vi "Acel_calib_detector.vi"(4 "Frecuencia\nmuestreo":dbl, 5 "Pattern frequency (Hz)":dbl, 6 "Nº canales":i32, 7 "All Files in Dir":path[](array[path])) -> (0 "Continue calibrating?":bool, 1 "Reporting":string, 2 "Acceler.\ndetected":i32, 3 "Acel Cal measurements":sgl[][](array[numeric]))   [LabVIEW 2015]
uses:
  <vilib>/measure/NI_MAPro.lvlib
  <vilib>/measure/madcrms.llb/Basic Averaged DC-RMS for 1 Chan.vi
  <vilib>/Analysis/NI_AALPro.lvlib
  <vilib>/Analysis/5stat.llb/RMS (DBL).vi
panel:
  out "size(s) 3":i32
  out "size(s) 2":i32[](array[numeric])
  out "size(s)":i32[](array[numeric])
  out "element":i32
  out "max index(es)":i32
  out "max value":i32
  out "Array 3":i32[](array[numeric])
  out "sorted array":i32[](array[numeric])
  out "Array":i32[](array[numeric])
  out "OK files":bool[](array[boolean])
  out "Nº meas":i32
  out "Valid\nindex":i32[](array[numeric])
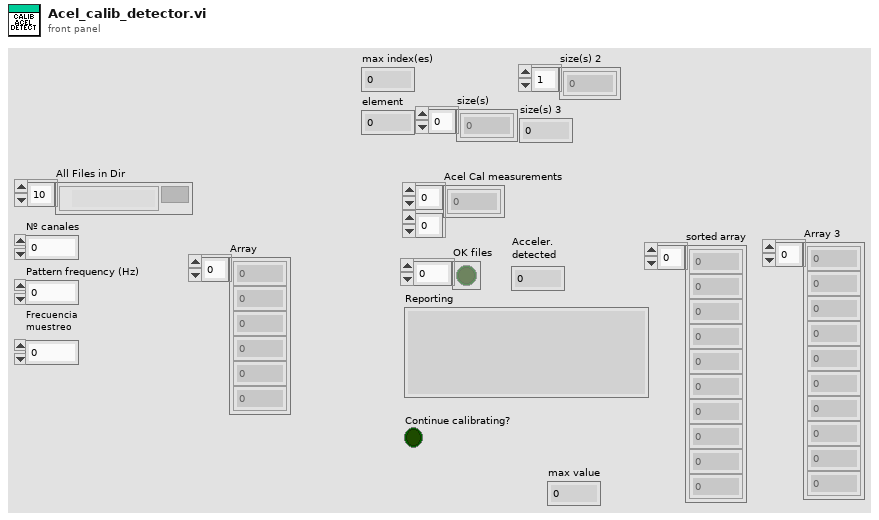
[diagram p1: front panel]
types:
  T1 = enum16{"big-endian, network order", "native, host order", "little-endian"}
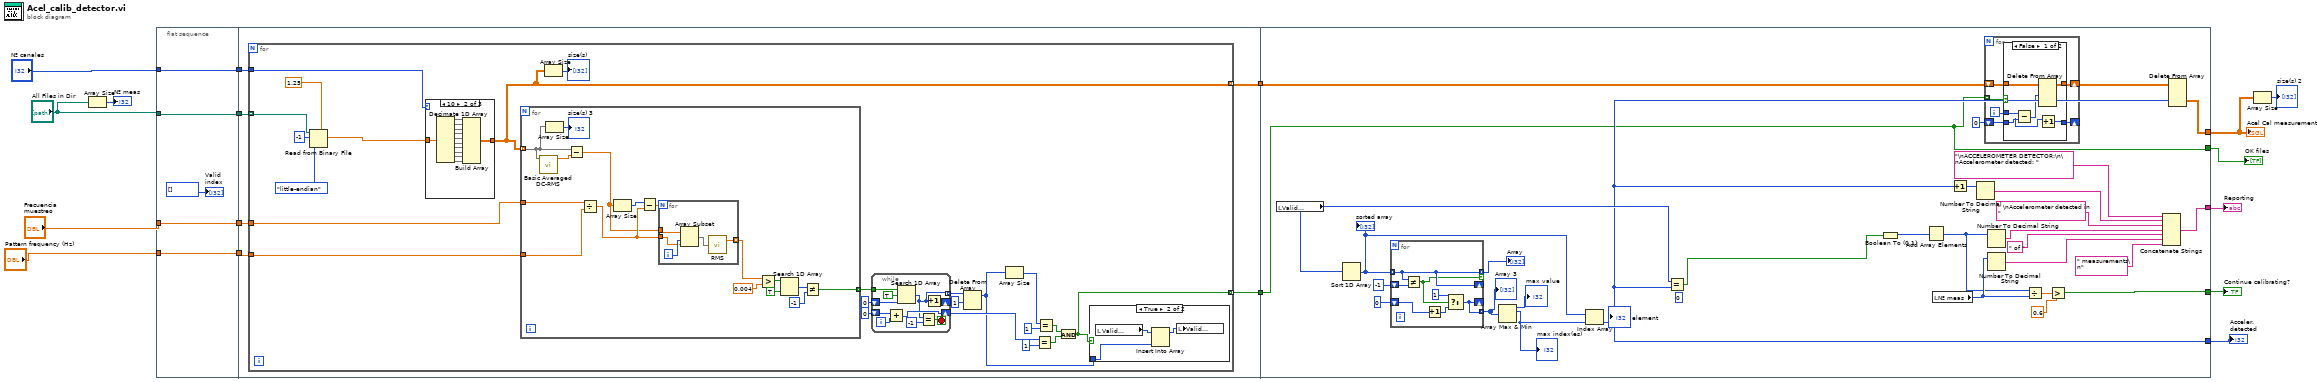
[diagram p0: block diagram]
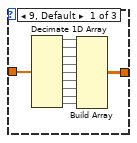
[diagram p3: hidden frame]
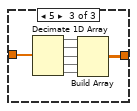
[diagram p4: hidden frame]
diagram:
  n1 = Array Size(array="All Files in Dir") -> (size(s)=→"Nº meas":i32)
  n2 = flat-sequence {
    tunnel: "All Files in Dir" -> [w21]
    tunnel: [w21] -> w17
    tunnel: [w20] -> w16
    tunnel: "Nº canales" -> [w20]
    tunnel: [w19] -> w15
    tunnel: "Frecuencia\nmuestreo" -> [w19]
    tunnel: [w18] -> w14
    tunnel: "Pattern frequency (Hz)" -> [w18]
    tunnel: [w27] -> w13
    tunnel: [w26] -> w12
    tunnel: w17 -> [w28]
    tunnel: w16 -> [w25]
    tunnel: w15 -> [w24]
    tunnel: w14 -> [w23]
    tunnel: w13 -> [w116]
    tunnel: w12 -> [w142]
    tunnel: [w141] -> w2
    tunnel: [w135] -> w4
    tunnel: [w116] -> w6
    tunnel: [w134] -> w5
    tunnel: [w121] -> w3
    frame #0 {
      "Valid\nindex" <- i32[] []
    }
    frame #1 {
      n3 = for {
        tunnel: w28 -> [w47] mode=indexing
        tunnel: [w37] -> w27 mode=indexing
        tunnel: [w30] -> w26 mode=indexing
        tunnel: w25 -> [w35]
        tunnel: w24 -> [w34]
        tunnel: w23 -> [w33]
        n4 = Read from Binary File(5:sgl 1.25, 9:T1."little-endian" ("byte order (0:big-endian, network order)"), 10:-1 ("count (1)"), 11:w47) -> (2:w48:sgl[])  [unwired: 1 in, 4 out]
        n5 = case shown="10" w35 {
          tunnel: [w65 w78 w88] -> w30
          tunnel: w48 -> [w66 w76 w89]
          frame 9, Default {
            n6 = Decimate 1D Array(w66) -> (w67:sgl[], w75:sgl[], w74:sgl[], w70:sgl[], w69:sgl[], w71:sgl[], w72:sgl[], w73:sgl[], w68:sgl[])
            n7 = Build Array(w67, w75, w74, w70, w69, w71, w72, w73, w68) -> (w65:sgl[][])
          }
          frame 10 {
            n8 = Decimate 1D Array(w76) -> (w77:sgl[], w87:sgl[], w86:sgl[], w82:sgl[], w81:sgl[], w83:sgl[], w84:sgl[], w85:sgl[], w80:sgl[], w79:sgl[])
            n9 = Build Array(w77, w87, w86, w82, w81, w83, w84, w85, w80, w79) -> (w78:sgl[][])
          }
          frame 5 {
            n10 = Decimate 1D Array(w89) -> (w90:sgl[], w94:sgl[], w93:sgl[], w92:sgl[], w91:sgl[])
            n11 = Build Array(w90, w94, w93, w92, w91) -> (w88:sgl[][])
          }
        }
        n12 = for {
          tunnel: w30 -> [w97] mode=indexing
          tunnel: [w100] -> w44 mode=indexing
          tunnel: w34 -> [w99]
          tunnel: w33 -> [w98]
          n13 = call-poly <vilib>:"Basic Averaged DC-RMS.vi"("signal in"=w97) -> ("DC value"=w110:dbl)  [unwired: 7 in, 3 out]
          n14 = Array Size(array=w97) -> (size(s)=→"size(s) 3":i32)
          n15 = Subtract(x=w97, y=w110) -> (x-y=w106:dbl[])
          n16 = Divide(x=w99, y=w98) -> (x/y=w107:dbl)
          n17 = Array Size(array=w106) -> (size(s)=w108:i32)
          n18 = Subtract(x=w108, y=w107) -> (x-y=w109:dbl)
          n19 = for {
            N: w109 -> [_]
            tunnel: w107 -> [w112]
            tunnel: [w115] -> w95 mode=indexing
            tunnel: w106 -> [w114]
            i -> [w113]
            n20 = Array Subset(array=w114, index=w113, length=w112) -> (w111:dbl[])
            n21 = call-poly <vilib>:"RMS.vi"("X"=w111) -> ("rms value"=w115:dbl)  [unwired: 1 out]
          }
          n22 = Greater?(x=w95, y=0.004 ("threshold y")) -> (0:w104:bool[])
          n23 = Search 1D Array(1D array=w104, element=TRUE) -> (index of element=w102:i32)  [unwired: 1 in]
          n24 = Not Equal?(x=w102, y=-1) -> (x != y?=w100:bool)
        }
        n25 = Array Size(array=w30) -> (size(s)=→"size(s)":i32[])
        n26 = while {
          tunnel: w44 -> [w64]
          shift-right: [w56] -> _
          shift-left: 0 ("index of element") -> [w61]
          shift-right: [w57] -> w36
          shift-left: 0 ("index of element") -> [w58]
          tunnel: [w55] -> w32 mode=indexing
          i -> [w59]
          stop <- w62 stop-if-true
          n27 = Add(x=w58, y=w59) -> (x+y=w57:i32)
          n28 = Search 1D Array(1D array=w64, element=TRUE, start index (0)=w61) -> (index of element=w55:i32)
          n29 = Equal?(x=w55, y=-1) -> (x = y?=w62:bool)
          n30 = Increment(x=w55) -> (x+1=w56:i32)
        }
        n31 = Delete From Array(array=w32, length=1) -> (array with subset deleted=w31:i32[])  [unwired: 1 in, 1 out]
        n32 = Array Size(array=w31) -> (size(s)=w40:i32)
        n33 = Equal?(x=w36, y=1) -> (x = y?=w39:bool)
        n34 = Equal?(x=w40, y=1) -> (x = y?=w38:bool)
        n35 = And(x=w38, y=w39) -> (x .and. y?=w37:bool)
        n36 = case shown="True" w37 {
          tunnel: w31 -> [_ w54]
          frame False {
          }
          frame True {
            n37 = local read "Valid\nindex"() -> (w52:i32[])
            n38 = Insert Into Array(array=w52, new element=w54) -> (w53:i32[])  [unwired: 1 in]
            n39 = local write "Valid\nindex"(w53) -> ()
          }
        }
      }
    }
    frame #2 {
      (unwired) 0 ("index of element")
      n40 = local read "Valid\nindex"() -> (w123:i32[])
      n41 = Sort 1D Array(array=w123) -> (sorted array=w117:i32[])
      "sorted array" <- w117
      n42 = for {
        tunnel: w117 -> [w151] mode=indexing
        shift-right: [w151] -> _
        shift-left: -1 ("y") -> [w152]
        tunnel: [w151] -> w128 mode=indexing if=w150
        shift-right: [w147] -> _
        shift-left: 0 ("y") -> [w148]
        tunnel: [w147] -> w126 mode=indexing
        n43 = Not Equal?(x=w151, y=w152) -> (x != y?=w150:bool)
        n44 = Increment(x=w148) -> (x+1=w149:i32)
        n45 = Select(t=1 ("y"), s=w150, f=w149) -> (s? t:f=w147:i32)
      }
      "Array" <- w128
      "Array 3" <- w126
      n46 = Array Max & Min(array=w126) -> (max value=→"max value":i32, max index (indices)=w124:i32)  [unwired: 2 out]
      "max index(es)" <- w124
      n47 = Index Array(array=w117, index=w124) -> (element=w121:i32)
      "element" <- w121
      n48 = Equal?(x=w123, y=w121) -> (x = y?=w120:bool[])
      n49 = Boolean To (0,1)(Boolean=w120) -> (0, 1=w119:i16[])
      n50 = Add Array Elements(numeric array=w119) -> (sum=w118:i16)
      n51 = local read "Nº meas"() -> (w136:i32)
      n52 = Increment(x=w121) -> (x+1=w122:i32)
      n53 = Number To Decimal String(number=w122) -> (decimal integer string=w132:string)  [unwired: 1 in]
      n54 = for {
        tunnel: w116 -> [w157] mode=indexing
        shift-right: [w156] -> w140
        shift-left: w142 -> [w158]
        shift-right: [w153] -> _
        shift-left: 0 ("index of element") -> [w154]
        i -> [w155]
        n55 = case shown="False" w157 {
          tunnel: w158 -> [w164 w166]
          tunnel: [w163 w166] -> w156
          tunnel: w155 -> [w162 _]
          tunnel: w154 -> [w159 w165]
          tunnel: [w160 w165] -> w153
          frame False {
            n56 = Subtract(x=w162, y=w159) -> (x-y=w161:i32)
            n57 = Delete From Array(array=w164, index (dim 0)=w161) -> (array with subset deleted=w163:sgl[][][])  [unwired: 3 in, 1 out]
            n58 = Increment(x=w159) -> (x+1=w160:i32)
          }
          frame True {
          }
        }
      }
      n59 = Number To Decimal String(number=w118) -> (decimal integer string=w145:string)  [unwired: 1 in]
      n60 = Number To Decimal String(number=w136) -> (decimal integer string=w143:string)  [unwired: 1 in]
      n61 = Divide(x=w118, y=w136) -> (x/y=w138:dbl)
      n62 = Greater?(x=w138, y=0.6) -> (0:w135:bool)
      n63 = Concatenate Strings("\nACCELEROMETER DETECTOR:\n\nAccelerometer detected: ", w132, " \nAccelerometer detected in  ", w145, " of ", w143, " measurements\n") -> (w134:string)
      n64 = Delete From Array(array=w140, index (dim 1)=w121) -> (deleted portion=w141:sgl[][])  [unwired: 3 in, 1 out]
    }
  }
  n65 = Array Size(array=w2) -> (size(s)=→"size(s) 2":i32[])
  "Acel Cal measurements" <- w2
  "OK files" <- w6
  "Reporting" <- w5
  "Continue calibrating?" <- w4
  "Acceler.\ndetected" <- w3
